vi "XY Graph Tipstrip Mouse Enter.vi"(8 "Error In":errorcluster, 10 "Event Registration Refnum":refnum<event-registration>, 11 "XY Graph Refnum":T1) -> (0 "Error Out":errorcluster, 2 "Event Registration Refnum":refnum<event-registration>)   [LabVIEW 2021, in "XY Graph Add-Ons.lvlib"]
doc: "Connect the corresponding dynamic event clusters of the Event Structure's \"Mouse Enter\" event for the XYGraph to this subVI"
uses:
  XY Graph/XY Graph Add-Ons.lvlib
  XY Graph/XY Graph Refnum.ctl
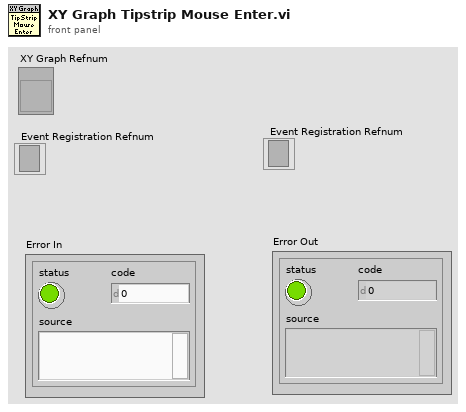
[diagram p1: front panel]
types:
  T1 = typedef "XY Graph Add-Ons.lvlib/XY Graph Refnum.ctl" = refnum<vi>
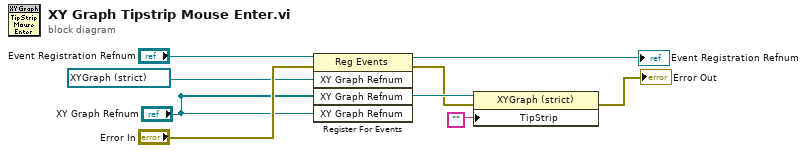
[diagram p0: block diagram]
diagram:
  n1 = register-events(reference="Event Registration Refnum", error in="Error In", refnum<vi> refnum ("event source"), "XY Graph Refnum", "XY Graph Refnum") -> (reference out=→"Event Registration Refnum":refnum<event-registration>, error out=w2:errorcluster)
  n2 = property class="XYGraph (strict)"(reference="XY Graph Refnum", error in=w2, "TipStrip"="") -> (error out=→"Error Out":errorcluster)  [unwired: 1 out]
